vi "test_serialize_deserialize.vi"() -> ()   [LabVIEW 2020, in "NI_ADAS_IMAQ_Array.lvlib"]
doc: "Version 0.1"
uses:
  NI_ADAS_IMAQ_Array.lvlib
  Process Data.ctl
  <vilib>/vision/Image Controls.llb/IMAQ Image.ctl
  Serialize Data.vi
  Deserialize Data.vi
  Serialize Data.vi/69b4f655-d322-486f-8d65-ee31f7d8c6ef.vi
  Deserialize Data.vi/5e2451cd-7b8c-4079-9add-41a600a01e16.vi
  <vilib>/ADAS Record/IODataPEF/Error/Error_CheckAndSetDllError.vi
  <vilib>/ADAS Record/IODataPEF/Error/Error_SetError.vi
  <vilib>/ADAS Record/IODataPEF/CfgMgr/GetPEFConfiguration_DefaultFlatFormat.vi
  <vilib>/ADAS Record/IODataPEF/Error/ErrorMgr.vi
  <vilib>/ADAS Record/CustomData/_Custom_RegisterType.vi
  <vilib>/addons/_JKI Toolkits/Caraya/classes/Test/Test.lvclass
  <vilib>/addons/_JKI Toolkits/Caraya/classes/Assert/Assert.lvclass
panel:
  out "serialized image":T1(plugin-control)
  out "original image":T1(plugin-control)
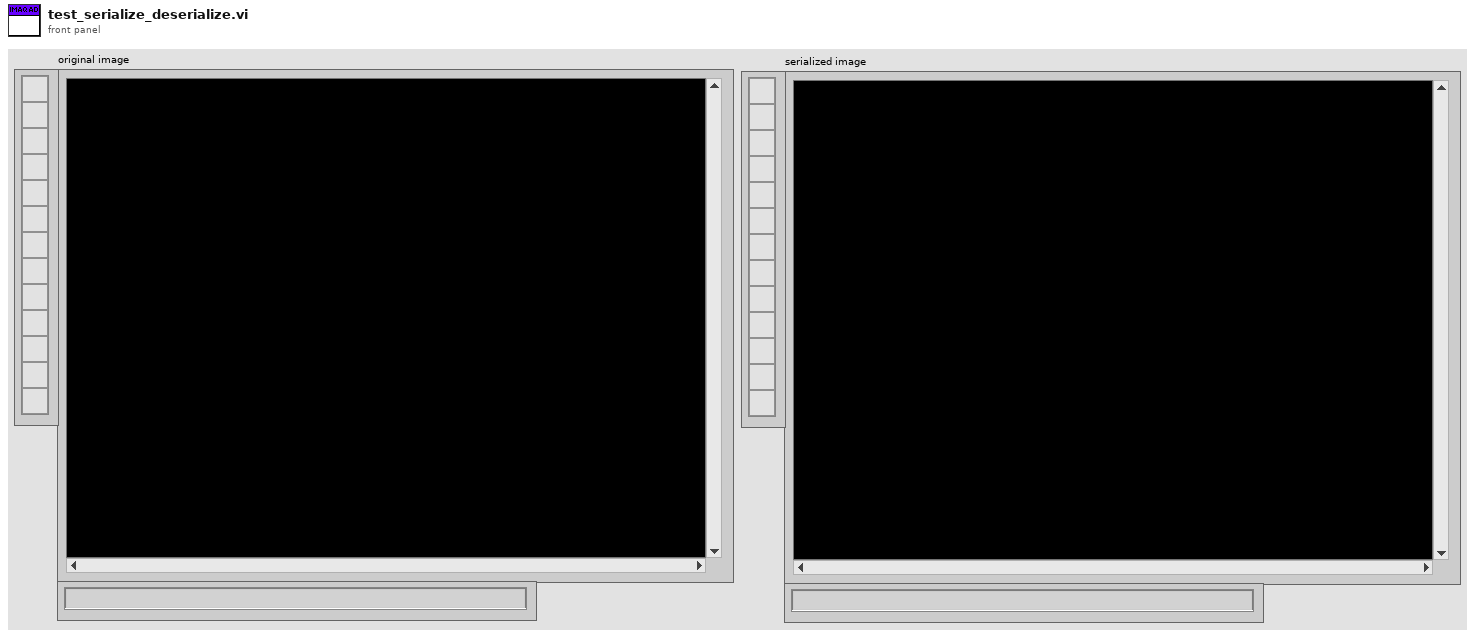
[diagram p1: front panel]
types:
  T1 = typedef "IMAQ Image.ctl" = refnum<image>
  T2 = typedef "NI_ADAS_IMAQ_Array.lvlib/Process Data.ctl" = cluster{"Timestamp":timestamp, "Bus Channel":u16, "Image Array":T1[]}
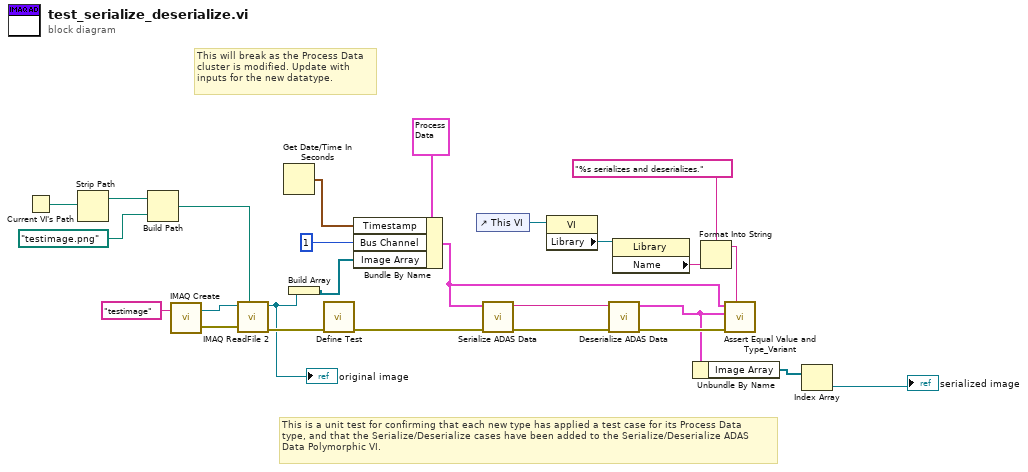
[diagram p0: block diagram]
diagram:
  # "This will break as the Process Data\ncluster is modified. Update with\ninputs for the new datatype."
  # "This is a unit test for confirming that each new type has applied a test case for its Process Data\ntype, and that the Serialize/Deserialize cases have been added to the Serialize/Deserialize ADAS\nData Polymorphic VI."
  n1 = Current VI's Path() -> (path=w11:path)
  n2 = Strip Path(path=w11) -> (stripped path=w10:path)  [unwired: 1 out]
  n3 = Build Path(base path=w10, name or relative path=path "testimage.png") -> (appended path=w8:path)
  n4 = call "IMAQ Create"("Image Name"="testimage") -> ("New Image"=w13:T1, "error out"=w12:errorcluster)  [unwired: 4 in]
  n5 = call "IMAQ ReadFile 2"("File Path"=w8, "error in (no error)"=w12, "Image"=w13) -> ("error out"=w6:errorcluster, "Image Out"=w2:T1)  [unwired: 4 in, 3 out]
  "original image" <- w2
  n6 = Get Date/Time In Seconds() -> (seconds since 1Jan1904=w16:timestamp)
  n7 = Build Array(w2) -> (w7:T1[])
  n8 = call <vilib>:"Define Test.vi"("error in (no error)"=w6) -> ("error out"=w21:errorcluster)  [unwired: 10 in]
  n9 = Bundle By Name(cluster=T2 {"Timestamp"=timestamp(0 s since 1904-01-01), "Bus Channel"=0, "Image Array"=[]} ("Process Data in"), "Timestamp"=w16, "Bus Channel"=u16 1, "Image Array"=w7) -> (w5:T2)
  n10 = control-ref of="This VI"() -> (w26:refnum<vi>)
  n11 = call-poly "Serialize ADAS Data.vi"("error in (no error)"=w21, "Process Data"=w5) -> ("error out"=w20:errorcluster, "Flat Data out"=w19:string)  [unwired: 8 in]
  n12 = property class="VI"(reference=w26) -> ("Library"=w25:refnum<vi>)  [unwired: 1 in, 2 out]
  n13 = call-poly "Deserialize ADAS Data.vi"("error in (no error)"=w20, "Flat Data in"=w19) -> ("error out"=w18:errorcluster, "Process Data out"=w4:T2)  [unwired: 8 in]
  n14 = property class="Library"(reference=w25) -> ("Name"=w23:string)  [unwired: 1 in, 2 out]
  n15 = Unbundle By Name(w4) -> ("Image Array"=w3:T1[])
  n16 = Format Into String(format string="%s serializes and deserializes.", w23) -> (resulting string=w22:string)  [unwired: 2 in, 1 out]
  n17 = call <vilib>:"Assert Equal Value and Type_Variant.vi"("Label"=w22, "error in (no error)"=w18, "Y"=w4, "X"=w5) -> ()  [unwired: 7 in, 1 out]
  n18 = Index Array(array=w3) -> (element=→"serialized image":T1)  [unwired: 1 in]
